vi "RTS Shutdown.vi"(7 "Stop Event":refnum<user-event>, 8 "error in":errorcluster) -> (0 "error out":errorcluster)   [LabVIEW 2020]
uses:
  PCT FGV CMD.ctl
  User Event - Stop/User Event - Stop.lvlib
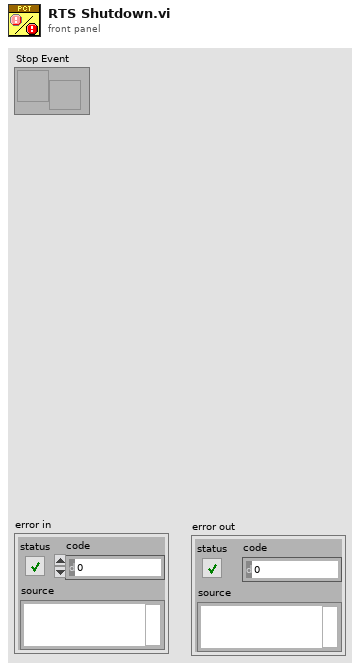
[diagram p1: front panel]
types:
  T1 = typedef "PCT FGV CMD.ctl" = enum16{"INIT", "GET", "SET"}
  T2 = typedef "Message Queue.lvlib/All Message Queues.ctl" = cluster{"UI":refnum<queue>, "Logging":refnum<queue>, "LOG":refnum<queue>, "ALARM":refnum<queue>, "Test":refnum<queue>, "Answer":refnum<queue>, "PLC":refnum<queue>, "DB":refnum<queue>, "Report":refnum<queue>, "OPC":refnum<queue>, "Procedure":refnum<queue>, "PalmSens":refnum<queue>, "SYS 7000 Reader":refnum<queue>, "SWITCH":refnum<queue>, "MOTOR":refnum<queue>, "MOTION":refnum<queue>, "HIDEN":refnum<queue>, "VALVE":refnum<queue>, "MFC":refnum<queue>, "PUMP IN":refnum<queue>, "PUMP OUT":refnum<queue>}
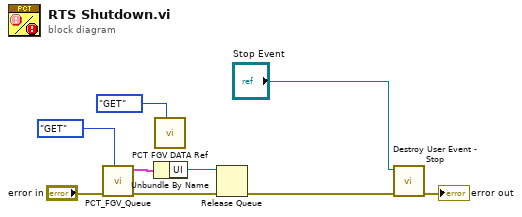
[diagram p0: block diagram]
diagram:
  n1 = call "PCT_FGV_Queue.vi"("CMD"=PCT_FGV_CMD."GET", "error in (no error)"="error in") -> ("error out"=w1:errorcluster, "Message Queues out"=w3:T2)  [unwired: 8 in]
  n2 = Unbundle By Name(w3) -> ("UI"=w2:refnum<queue>)
  n3 = call "PCT FGV DATA Ref.vi"("CMD"=PCT_FGV_CMD."GET") -> ()  [unwired: 9 in, 2 out]
  n4 = Release Queue(queue=w2, error in (no error)=w1) -> (error out=w8:errorcluster)  [unwired: 1 in, 2 out]
  n5 = call "Destroy User Event - Stop.vi"("error in (no error)"=w8, "User Event - Stop"="Stop Event") -> ("error out"=→"error out":errorcluster)  [unwired: 9 in]
